vi "LVAPT-GIT-Pull.vi"(11 "path":path) -> ()   [LabVIEW 2019]
uses:
  <vilib>/Hampel Software Engineering/Git API/Git API/GIT-api.lvclass/GIT-api.ctl
  <vilib>/Hampel Software Engineering/Git API/Git API/Accessors/GIT-Set Working Dir.vi
  <vilib>/Hampel Software Engineering/Git API/Git API/GIT-api.lvclass
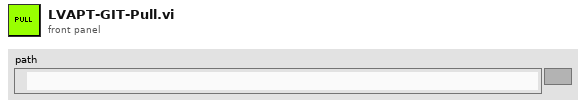
[diagram p1: front panel]
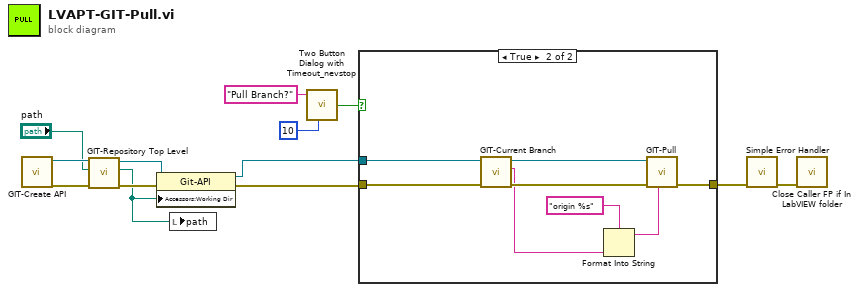
[diagram p0: block diagram]
diagram:
  n1 = call <vilib>:"GIT-Create API.vi"() -> ("error out"=w10:errorcluster, "git-api out"=w11:refnum<class "GIT-api.lvclass">)  [unwired: 10 in]
  n2 = call <vilib>:"GIT-Repository Top Level.vi"("error in"=w10, "Current Path"="path", "git-api in"=w11) -> ("error out"=w13:errorcluster, "Repo Top Level Path"=w1:path, "git-api out"=w12:refnum<class "GIT-api.lvclass">)  [unwired: 6 in]
  n3 = property class="Git-API"(reference=w12, error in=w13, "Accessors:Working Dir"=w1) -> (reference out=w8:refnum<class "GIT-api.lvclass">, error out=w9:errorcluster)
  n4 = local write "path"(w1) -> ()
  n5 = call <userlib>:"Two Button Dialog with Timeout_nevstop.vi"("message"="Pull Branch?", "F Timeout(-1 s)"=10) -> ("T button?"=w4:bool)  [unwired: 3 in]
  n6 = case shown="True" w4 {
    tunnel: w9 -> [w14 w20]
    tunnel: [w14 w22] -> w3
    tunnel: w8 -> [_ w21]
    frame False {
    }
    frame True {
      n7 = call <vilib>:"GIT-Current Branch.vi"("error in"=w20, "git-api in"=w21) -> ("error out"=w18:errorcluster, "current branch"=w15:string, "git-api out"=w19:refnum<class "GIT-api.lvclass">)  [unwired: 7 in]
      n8 = Format Into String(format string="origin %s" ("param"), w15) -> (resulting string=w16:string)  [unwired: 2 in, 1 out]
      n9 = call <vilib>:"GIT-Pull.vi"("param"=w16, "error in"=w18, "git-api in"=w19) -> ("error out"=w22:errorcluster)  [unwired: 7 in, 1 out]
    }
  }
  n10 = call <vilib>:"Simple Error Handler.vi"("error in (no error)"=w3) -> ("error out"=w2:errorcluster)  [unwired: 4 in, 4 out]
  n11 = call "Close Caller FP if In LabVIEW folder.vi"("error in (no error)"=w2) -> ()  [unwired: 10 in, 1 out]
